vi "Read.vi"(8 "error in (no error)":errorcluster, 10 "response size":u8=2, 11 "VISA resource name":refnum<visa-resource-name>) -> (0 "error out":errorcluster, 2 "response array":u8[](array[numeric]), 3 "VISA resource name out":refnum<visa-resource-name>)   [LabVIEW 2017, in "Digikrom DK24x.lvlib"]
doc: "Reads the number of bytes specified by 'response size' from the VISA resource"
uses:
  Digikrom DK24x.lvlib
panel:
  out "Response":string
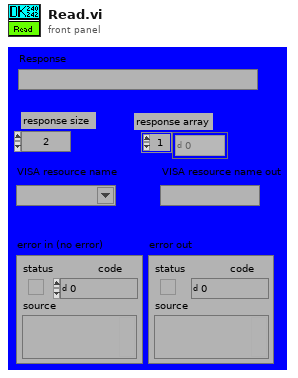
[diagram p1: front panel]
types:
  T1 = typedef "Semaphore RefNum" = refnum<k1>
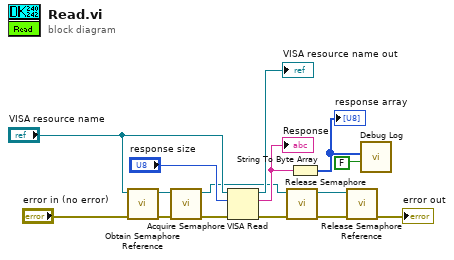
[diagram p0: block diagram]
diagram:
  n1 = call <vilib>:"Obtain Semaphore Reference.vi"("error in (no error)"="error in (no error)", "name (unnamed)"="VISA resource name") -> ("error out"=w9:errorcluster, "semaphore"=w8:T1)  [unwired: 3 in, 1 out]
  n2 = call <vilib>:"Acquire Semaphore.vi"("error in (no error)"=w9, "semaphore"=w8) -> ("error out"=w6:errorcluster, "semaphore out"=w5:T1)  [unwired: 3 in, 1 out]
  n3 = VISA Read(VISA resource name="VISA resource name", byte count="response size", error in (no error)=w6) -> (VISA resource name out=→"VISA resource name out":refnum<visa-resource-name>, read buffer=w13:string, error out=w4:errorcluster)  [unwired: 1 out]
  "Response" <- w13
  n4 = call <vilib>:"Release Semaphore.vi"("error in (no error)"=w4, "semaphore"=w5) -> ("error out"=w2:errorcluster, "semaphore out"=w3:T1)  [unwired: 4 in]
  n5 = String To Byte Array(string=w13) -> (unsigned byte array=w12:u8[])
  "response array" <- w12
  n6 = call <vilib>:"Release Semaphore Reference.vi"("error in (no error)"=w2, "semaphore"=w3) -> ("error out"=→"error out":errorcluster)  [unwired: 8 in, 1 out]
  n7 = call "Debug Log.vi"("Write?"=FALSE, "Data"=w12) -> ()  [unwired: 1 in, 9 out]
